vi "MTS_ToImageOffline.vi"(0 "Data In":u32[](array[numeric]), 1 "Reset":bool, 2 "Image Array In":i32[][](array[numeric]), 5 "Data Count":i32, 9 "Pixel Time (Laser Pulses)":i32, 11 "Trace Bins":i32=25) -> (3 "Image Array Out":i32[][](array[numeric]), 4 "Histograms":i32[][](array[numeric]), 6 "Total Photon Count":u64[](array[numeric]), 8 "Trigger Times":u64[](array[numeric]), 13 "Total Oveflow Count":u64, 14 "Num Records Total":i32, 15 "Traces":i32[][](array[numeric]))   [LabVIEW 2011]
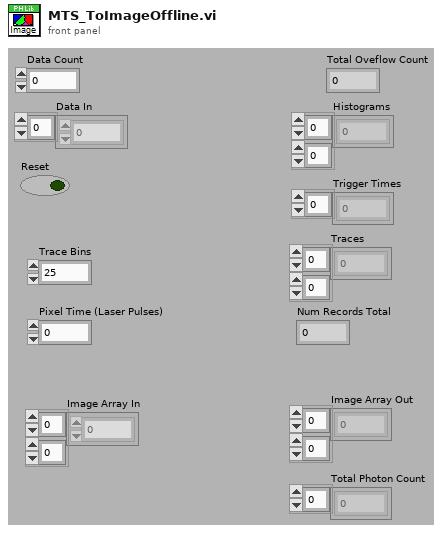
[diagram p1: front panel]
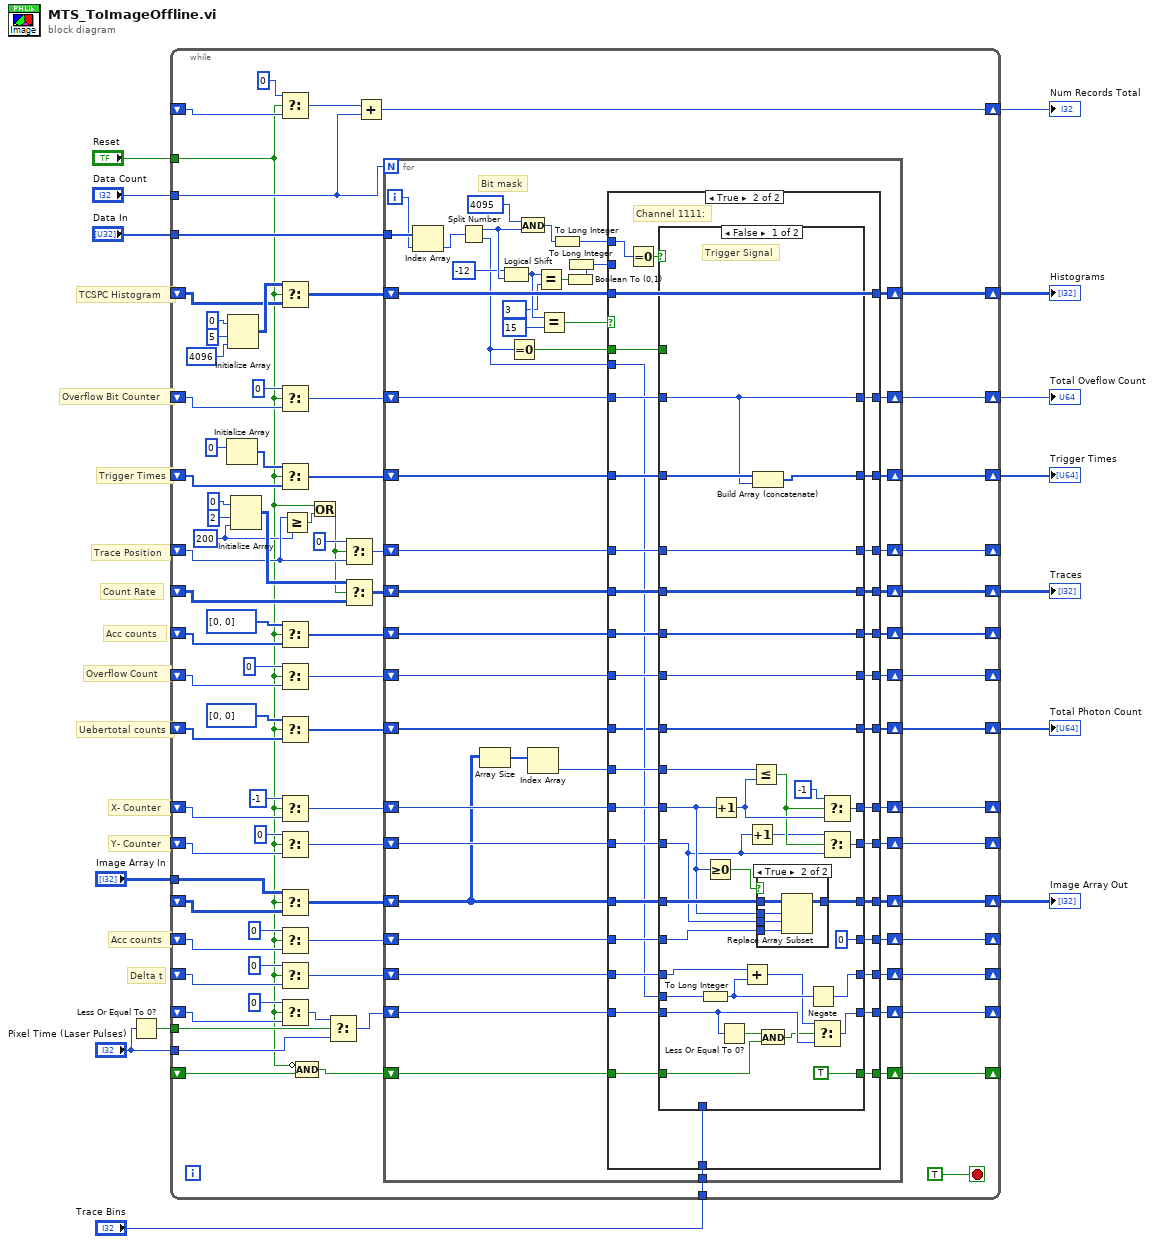
[diagram p0: block diagram]
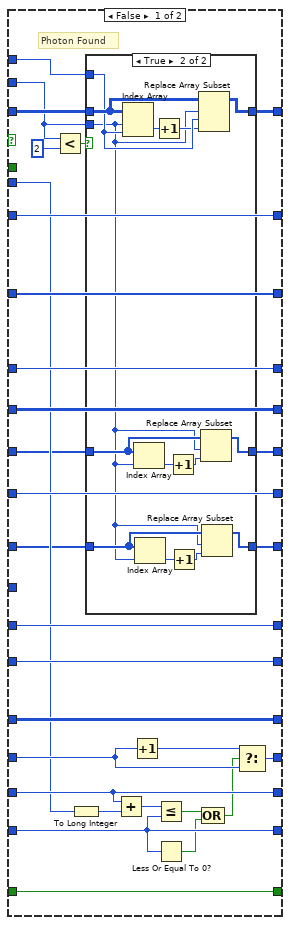
[diagram p2: hidden frame]
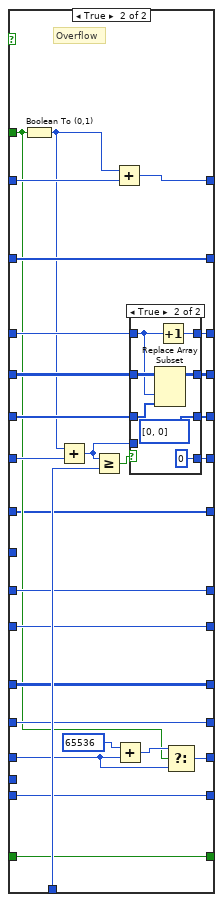
[diagram p5: hidden frame]
diagram:
  # "Uebertotal counts"
  # "Y- Counter"
  # "X- Counter"
  # "Delta t"
  # "Acc counts"
  # "Trace Position"
  # "Overflow Count"
  # "Acc counts"
  # "Count Rate"
  # "Trigger Times"
  # "TCSPC Histogram"
  # "Overflow Bit Counter"
  n1 = Less Or Equal To 0?(x="Pixel Time (Laser Pulses)") -> (x <= 0?=w2:bool)
  n2 = while {
    tunnel: "Data In" -> [w92]
    shift-right: [w93] -> w14
    shift-left: _ -> [w88]
    tunnel: "Reset" -> [w15]
    shift-right: [w85] -> w4
    shift-left: _ -> [w84]
    shift-right: [w80] -> w11
    shift-left: _ -> [w79]
    shift-right: [w75] -> w9
    shift-left: _ -> [w74]
    shift-right: [w72] -> _
    shift-left: _ -> [w71]
    shift-right: [w69] -> _
    shift-left: _ -> [w68]
    tunnel: "Trace Bins" -> [w67]
    shift-right: [w64] -> _
    shift-left: _ -> [w62]
    shift-right: [w58] -> w7
    shift-left: _ -> [w57]
    tunnel: "Image Array In" -> [w60]
    shift-right: [w53] -> _
    shift-left: _ -> [w51]
    shift-right: [w52] -> _
    shift-left: _ -> [w50]
    shift-right: [w45] -> _
    shift-left: _ -> [w43]
    shift-right: [w44] -> _
    shift-left: _ -> [w42]
    tunnel: "Data Count" -> [w37]
    shift-right: [w36] -> w5
    shift-left: _ -> [w39]
    shift-right: [w27] -> w3
    shift-left: _ -> [w26]
    shift-right: [w22] -> _
    shift-left: _ -> [w19]
    tunnel: w2 -> [w24]
    tunnel: "Pixel Time (Laser Pulses)" -> [w23]
    shift-right: [w18] -> _
    shift-left: _ -> [w17]
    stop <- TRUE stop-if-true
    w33 = 200 ("dimension size")
    n3 = Initialize Array(u64 0 ("element")) -> (w82:u64[])  [unwired: 1 out]
    n4 = Initialize Array(0 ("element"), 5 ("dimension size"), 4096 ("dimension size")) -> (w89:i32[][])
    n5 = Initialize Array(0 ("element"), 2 ("dimension size"), w33) -> (w77:i32[][])
    n6 = Select(t=0 ("Data Count 2"), s=w15, f=w39) -> (s? t:f=w38:i32)
    n7 = Select(t=w89, s=w15, f=w88) -> (s? t:f=w90:i32[][])
    n8 = Select(t=u64 0, s=w15, f=w84) -> (s? t:f=w86:u64)
    n9 = Select(t=w82, s=w15, f=w79) -> (s? t:f=w81:u64[])
    n10 = Select(t=u32[] [0, 0] ("initialized array"), s=w15, f=w71) -> (s? t:f=w73:u32[])
    n11 = Select(t=u32 0, s=w15, f=w68) -> (s? t:f=w70:u32)
    n12 = Select(t=u64[] [0, 0] ("initialized array"), s=w15, f=w26) -> (s? t:f=w28:u64[])
    n13 = Select(t=-1, s=w15, f=w43) -> (s? t:f=w47:i32)
    n14 = Select(t=0, s=w15, f=w42) -> (s? t:f=w46:i32)
    n15 = Select(t=w60, s=w15, f=w57) -> (s? t:f=w59:i32[][])
    n16 = Select(t=0, s=w15, f=w51) -> (s? t:f=w55:i32)
    n17 = Select(t=0, s=w15, f=w50) -> (s? t:f=w54:i32)
    n18 = Select(t=0, s=w15, f=w19) -> (s? t:f=w21:i32)
    n19 = Greater Or Equal?(x=w62, y=w33) -> (x >= y?=w63:bool)
    n20 = Compound Arithmetic op=AND(invert w15, w17) -> (w16:bool)
    n21 = Or(x=w15, y=w63) -> (x .or. y?=w61:bool)
    n22 = Select(t=w21, s=w24, f=w23) -> (s? t:f=w25:i32)
    n23 = Select(t=0, s=w61, f=w62) -> (s? t:f=w65:i32)
    n24 = Select(t=w77, s=w61, f=w74) -> (s? t:f=w76:i32[][])
    n25 = Add(x=w38, y=w37) -> (x+y=w36:i32)
    n26 = for {
      N: w37 -> [_]
      tunnel: w92 -> [w107]
      shift-right: [w140] -> w93
      shift-left: w90 -> [w142]
      shift-right: [w134] -> w85
      shift-left: w86 -> [w135]
      shift-right: [w132] -> w80
      shift-left: w81 -> [w133]
      shift-right: [w127] -> w75
      shift-left: w76 -> [w128]
      shift-right: [w129] -> w72
      shift-left: w73 -> [w130]
      shift-right: [w125] -> w69
      shift-left: w70 -> [w126]
      tunnel: w67 -> [w124]
      shift-right: [w122] -> w64
      shift-left: w65 -> [w123]
      shift-right: [w121] -> w58
      shift-left: w59 -> [w113]
      shift-right: [w119] -> w53
      shift-left: w55 -> [w120]
      shift-right: [w117] -> w52
      shift-left: w54 -> [w118]
      shift-right: [w114] -> w45
      shift-left: w47 -> [w115]
      shift-right: [w110] -> w44
      shift-left: w46 -> [w116]
      shift-right: [w98] -> w27
      shift-left: w28 -> [w99]
      shift-right: [w97] -> w22
      shift-left: w25 -> [w109]
      shift-right: [w96] -> w18
      shift-left: w16 -> [w95]
      i -> [w106]
      # "Bit mask"
      n27 = Index Array(array=w107, index=w106) -> (element=w105:u32)
      n28 = Split Number(x=w105) -> (hi(x)=w139:u16, lo(x)=w108:u16)
      n29 = Array Size(array=w113) -> (size(s)=w112:i32[])
      n30 = Logical Shift(y=i8 -12, x=w139) -> (x << y=w104:u16)
      n31 = Equal To 0?(x=w108) -> (x = 0?=w131:bool)
      n32 = And(x=u16 4095, y=w139) -> (x .and. y?=w143:u16)
      n33 = Index Array(array=w112) -> (element=w111:i32)  [unwired: 1 in]
      n34 = Equal?(x=w104, y=u16 3) -> (x = y?=w102:bool)
      n35 = Equal?(x=w104, y=u16 15) -> (x = y?=w136:bool)
      n36 = To Long Integer(number=w143) -> (32bit integer=w141:i32)
      n37 = Boolean To (0,1)(Boolean=w102) -> (0, 1=w101:i16)
      n38 = To Long Integer(number=w101) -> (32bit integer=w100:i32)
      n39 = case shown="True" w136 {
        tunnel: w142 -> [w174 w223]
        tunnel: w141 -> [w157 w204]
        tunnel: [w173 w223] -> w140
        tunnel: w100 -> [w153 _]
        tunnel: w135 -> [w172 w225]
        tunnel: [w172 w224] -> w134
        tunnel: w133 -> [w171 w222]
        tunnel: [w171 w221] -> w132
        tunnel: w131 -> [_ w220]
        tunnel: w130 -> [w156 w218]
        tunnel: [w155 w214] -> w129
        tunnel: w128 -> [w170 w217]
        tunnel: [w170 w213] -> w127
        tunnel: w126 -> [w169 w219]
        tunnel: [w169 w215] -> w125
        tunnel: w124 -> [_ w216]
        tunnel: w123 -> [w168 w212]
        tunnel: [w168 w211] -> w122
        tunnel: w113 -> [w167 w209]
        tunnel: [w167 w210] -> w121
        tunnel: w120 -> [w166 w205]
        tunnel: [w165 w206] -> w119
        tunnel: w118 -> [w164 w208]
        tunnel: [w164 w207] -> w117
        tunnel: w116 -> [w163 w203]
        tunnel: w115 -> [w162 w202]
        tunnel: [w162 w201] -> w114
        tunnel: w111 -> [_ w200]
        tunnel: [w163 w199] -> w110
        tunnel: w109 -> [w149 w195]
        tunnel: w108 -> [w159 w198]
        tunnel: w99 -> [w151 w197]
        tunnel: [w150 w196] -> w98
        tunnel: [w149 w194] -> w97
        tunnel: [w145 w193] -> w96
        tunnel: w95 -> [w145 w192]
        frame False {
          # "Photon Found"
          n40 = Less?(x=w153, y=2) -> (x < y?=w154:bool)
          n41 = To Long Integer(number=w159) -> (32bit integer=w158:i32)
          n42 = case shown="True" w154 {
            tunnel: w174 -> [w177 w191]
            tunnel: [w177 w190] -> w173
            tunnel: w157 -> [_ w189]
            tunnel: w153 -> [_ w178]
            tunnel: w156 -> [w176 w188]
            tunnel: [w176 w187] -> w155
            tunnel: w151 -> [w175 w180]
            tunnel: [w175 w179] -> w150
            frame False {
            }
            frame True {
              n43 = Index Array(array=w191, index (row)=w178, index (col)=w189) -> (element=w186:i32)
              n44 = Index Array(array=w188, index=w178) -> (element=w184:u32)
              n45 = Index Array(array=w180, index=w178) -> (element=w182:u64)
              n46 = Increment(x=w186) -> (x+1=w185:i32)
              n47 = Increment(x=w184) -> (x+1=w183:u32)
              n48 = Increment(x=w182) -> (x+1=w181:u64)
              n49 = Replace Array Subset(array=w191, new element=w185, index (row)=w178, index (col)=w189) -> (w190:i32[][])
              n50 = Replace Array Subset(array=w188, new element=w183, index=w178) -> (w187:u32[])
              n51 = Replace Array Subset(array=w180, new element=w181, index=w178) -> (w179:u64[])
            }
          }
          n52 = Add(x=w164, y=w158) -> (x+y=w160:i32)
          n53 = Increment(x=w166) -> (x+1=w161:i32)
          n54 = Less Or Equal?(x=w160, y=w149) -> (x <= y?=w148:bool)
          n55 = Less Or Equal To 0?(x=w149) -> (x <= 0?=w147:bool)
          n56 = Compound Arithmetic op=OR(w148, w147) -> (w146:bool)
          n57 = Select(t=w161, s=w146, f=w166) -> (s? t:f=w165:i32)
        }
        frame True {
          # "Channel 1111:"
          n58 = Equal To 0?(x=w204) -> (x = 0?=w226:bool)
          n59 = case shown="False" w226 {
            tunnel: w225 -> [w257 w291]
            tunnel: [w257 w290] -> w224
            tunnel: w222 -> [w259 w292]
            tunnel: [w258 w292] -> w221
            tunnel: w220 -> [_ w269]
            tunnel: w219 -> [w256 w275]
            tunnel: w218 -> [w255 w286]
            tunnel: w217 -> [w254 w284]
            tunnel: w216 -> [_ w289]
            tunnel: [w256 w287] -> w215
            tunnel: [w255 w285] -> w214
            tunnel: [w254 w283] -> w213
            tunnel: w212 -> [w253 w282]
            tunnel: [w253 w281] -> w211
            tunnel: [w251 w280] -> w210
            tunnel: w209 -> [w252 w280]
            tunnel: w208 -> [w236 w270]
            tunnel: [w238 w271] -> w207
            tunnel: [0 ("t") w278] -> w206
            tunnel: w205 -> [w250 w278]
            tunnel: w198 -> [w235 _]
            tunnel: w203 -> [w240 w277]
            tunnel: w202 -> [w245 w276]
            tunnel: [w247 w276] -> w201
            tunnel: w200 -> [w246 _]
            tunnel: [w241 w277] -> w199
            tunnel: w197 -> [w237 w268]
            tunnel: [w237 w268] -> w196
            tunnel: w195 -> [w232 w267]
            tunnel: [w231 w267] -> w194
            tunnel: [TRUE w266] -> w193
            tunnel: w192 -> [w227 w266]
            frame False {
              # "Trigger Signal"
              n60 = To Long Integer(number=w235) -> (32bit integer=w234:i32)
              n61 = Greater Or Equal To 0?(x=w245) -> (x >= 0?=w248:bool)
              n62 = Increment(x=w245) -> (x+1=w244:i32)
              n63 = Less Or Equal To 0?(x=w232) -> (x <= 0?=w230:bool)
              n64 = Add(x=w236, y=w234) -> (x+y=w233:i32)
              n65 = Increment(x=w240) -> (x+1=w239:i32)
              n66 = Less Or Equal?(x=w246, y=w244) -> (x <= y?=w242:bool)
              n67 = Build Array (concatenate)(w259, w257) -> (w258:u64[])
              n68 = case shown="True" w248 {
                tunnel: w252 -> [w260 w265]
                tunnel: [w260 w264] -> w251
                tunnel: w250 -> [_ w263]
                tunnel: w240 -> [_ w262]
                tunnel: w245 -> [_ w261]
                frame False {
                }
                frame True {
                  n69 = Replace Array Subset(array=w265, new element=w263, index (row)=w261, index (col)=w262) -> (w264:i32[][])
                }
              }
              n70 = And(x=w230, y=w227) -> (x .and. y?=w229:bool)
              n71 = Negate(x=w234) -> (-x=w238:i32)
              n72 = Select(t=w233, s=w229, f=w232) -> (s? t:f=w231:i32)
              n73 = Select(t=-1, s=w242, f=w244) -> (s? t:f=w247:i32)
              n74 = Select(t=w239, s=w242, f=w240) -> (s? t:f=w241:i32)
            }
            frame True {
              # "Overflow"
              n75 = Boolean To (0,1)(Boolean=w269) -> (0, 1=w273:i16)
              n76 = Add(x=w273, y=w275) -> (x+y=w274:u32)
              n77 = Greater Or Equal?(x=w274, y=w289) -> (x >= y?=w288:bool)
              n78 = Add(x=w273, y=w291) -> (x+y=w290:u64)
              n79 = Add(x=65536 ("t"), y=w270) -> (x+y=w272:i32)
              n80 = case shown="True" w288 {
                tunnel: w274 -> [w296 _]
                tunnel: [w296 u32 0] -> w287
                tunnel: w286 -> [w295 w301]
                tunnel: [w295 u32[] [0, 0] ("initialized array")] -> w285
                tunnel: w284 -> [w294 w302]
                tunnel: [w294 w300] -> w283
                tunnel: w282 -> [w293 w298]
                tunnel: [w293 w299] -> w281
                frame False {
                }
                frame True {
                  n81 = Replace Array Subset(array=w302, new element=w301, index (col)=w298) -> (w300:i32[][])  [unwired: 1 in]
                  n82 = Increment(x=w298) -> (x+1=w299:i32)
                }
              }
              n83 = Select(t=w272, s=w269, f=w270) -> (s? t:f=w271:i32)
            }
          }
        }
      }
    }
  }
  "Histograms" <- w14
  "Trigger Times" <- w11
  "Traces" <- w9
  "Image Array Out" <- w7
  "Num Records Total" <- w5
  "Total Oveflow Count" <- w4
  "Total Photon Count" <- w3
